vi "Prueba Instrument.vi"() -> ()   [LabVIEW 2020]
uses:
  Public/Controls/Motor initialization parameters--cluster.ctl
  Control de MaP.lvlib
panel:
  out "End":bool
  in  "Cluster":T1={"Action"=0, "Steps per rev motor 1"=0, "Steps per rev motor 2"=200, "RPM motor 1"=255, "RPM motor 2"=0, "Step style motor 1"=0, "Step style motor 2"=0} {"Step style motor 2" items=["Medio paso", "Paso completo"]; "Step style motor 1" items=["Medio paso", "Paso completo"]; "Action" items=["Unipolar", "Bipolar"]}
  in  "Enviar Datos":bool
  in  "Detener Procesos":bool
  out "Estado":string
  in  "Puerto Serial":refnum<visa-resource-name>
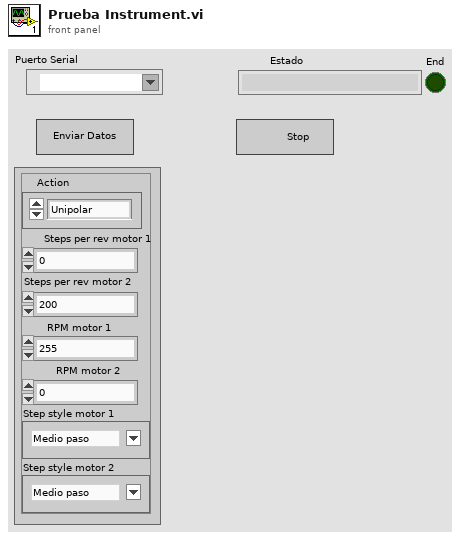
[diagram p1: front panel]
types:
  T1 = typedef "Control de MaP.lvlib/Motor initialization parameters--cluster.ctl" = cluster{"Action":u8, "Steps per rev motor 1":u16, "Steps per rev motor 2":u16, "RPM motor 1":u16, "RPM motor 2":u16, "Step style motor 1":u8, "Step style motor 2":u8}
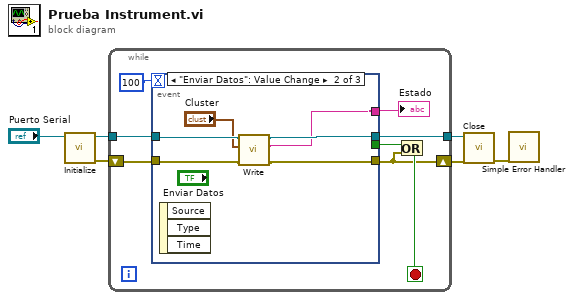
[diagram p0: block diagram]
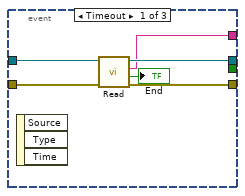
[diagram p2: hidden frame]
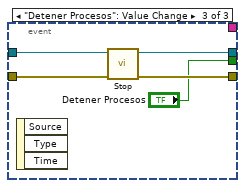
[diagram p3: hidden frame]
diagram:
  n1 = call "Initialize.vi"("Puerto Serial"="Puerto Serial") -> ("error out"=w4:errorcluster, "VISA resource name out"=w6:refnum<visa-resource-name>)  [unwired: 9 in]
  n2 = while {
    tunnel: w6 -> [w14]
    tunnel: [w13] -> w2
    shift-right: [w9] -> w3
    shift-left: w4 -> [w8]
    stop <- w11 stop-if-true
    n3 = event shown="[1] \"Enviar Datos\": Value Change" {
      selector: _ -> [_ _ _]
      dyn-events: _ -> [_ _ _]
      timeout: 100 -> [_ _ _]
      tunnel: w14 -> [w20 w22 w31]
      tunnel: w8 -> [w19 w23 w28]
      tunnel: [w18 w26 w30] -> w13
      tunnel: [w17 w24 w29] -> w9
      tunnel: [w16 w25 _] -> w12
      tunnel: [_ _ "Detener Procesos"] -> w7
      event Timeout {
        n4 = event-data() -> ()  [unwired: 1 in, 3 out]
        n5 = call "Read.vi"("error in (no error)"=w19, "VISA resource name"=w20) -> ("error out"=w17:errorcluster, "End"=→"End":bool, "Recibo de Datos"=w16:string, "VISA resource name out"=w18:refnum<visa-resource-name>)  [unwired: 6 in]
      }
      event "Enviar Datos": Value Change {
        n6 = event-data() -> ()  [unwired: 1 in, 3 out]
        n7 = call "Write.vi"("error in (no error)"=w23, "Comando"="Cluster", "VISA resource name"=w22) -> ("error out"=w24:errorcluster, "Comando(string)"=w25:string, "VISA resource name out"=w26:refnum<visa-resource-name>)  [unwired: 6 in]
      }
      event "Detener Procesos": Value Change {
        n8 = event-data() -> ()  [unwired: 1 in, 3 out]
        n9 = call "Stop.vi"("error in (no error)"=w28, "VISA resource name"=w31) -> ("error out"=w29:errorcluster, "VISA resource name out"=w30:refnum<visa-resource-name>)  [unwired: 8 in]
      }
    }
    "Estado" <- w12
    n10 = Or(x=w7, y=w9) -> (x .or. y?=w11:bool)
  }
  n11 = call "Close.vi"("error in (no error)"=w3, "VISA resource name"=w2) -> ("error out"=w1:errorcluster)  [unwired: 9 in]
  n12 = call <vilib>:"Simple Error Handler.vi"("error in (no error)"=w1) -> ()  [unwired: 4 in, 5 out]
